vi "Hysteresis-CalculateLinearPosition.vi"(9 "BWD/FWD":T2, 10 "hypothesis":T3(ring)=enum."middle", 11 "relative Range":dbl=1.0) -> (1 "LinBwdFwd":T1)   [LabVIEW 2016]
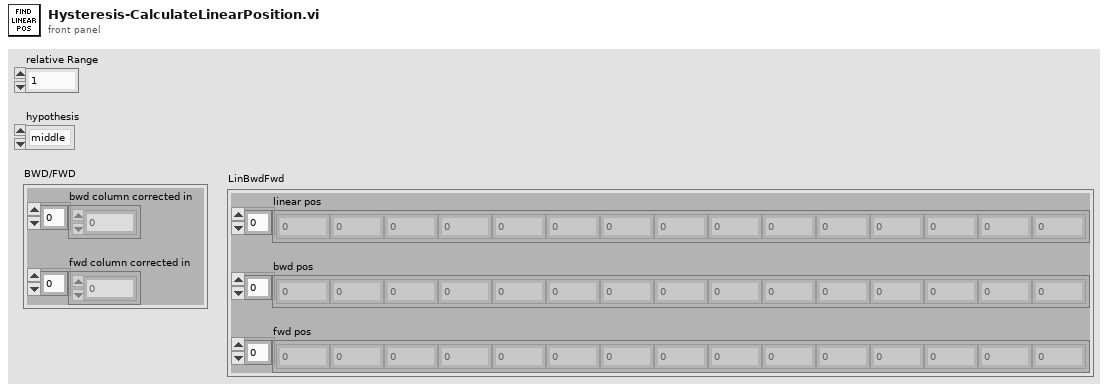
[diagram p1: front panel]
types:
  T1 = cluster{"linear pos ":dbl[], "bwd pos":dbl[], "fwd pos":dbl[]}
  T2 = cluster{"bwd column corrected in":dbl[], "fwd column corrected in":dbl[]}
  T3 = enum16{"bwd", "middle", "fwd", "linear", "2nd esti"}
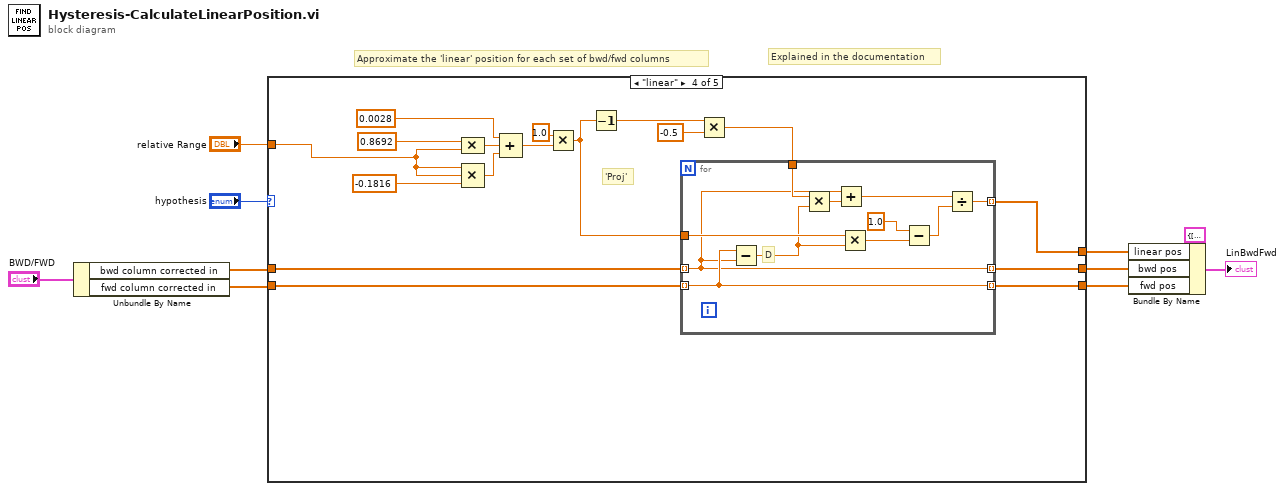
[diagram p0: block diagram]
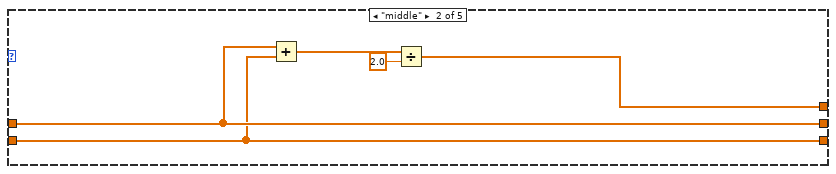
[diagram p3: hidden frame]
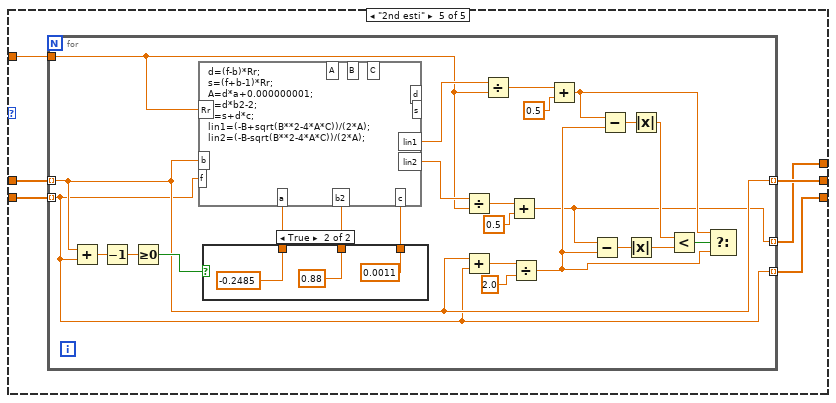
[diagram p5: hidden frame]
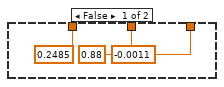
[diagram p6: hidden frame]
diagram:
  # "Explained in the documentation"
  # "Approximate the 'linear' position for each set of bwd/fwd columns"
  n1 = Unbundle By Name("BWD/FWD") -> ("bwd column corrected in"=w6:dbl[], "fwd column corrected in"=w7:dbl[])
  n2 = case shown="\"linear\"" "hypothesis" {
    tunnel: [w11 w14 w19 w36 w48] -> w5
    tunnel: [w12 w16 w19 w34 w50] -> w3
    tunnel: w6 -> [w11 w17 w18 w32 w52]
    tunnel: w7 -> [w12 w16 w19 w33 w53]
    tunnel: [w11 w17 w18 w35 w49] -> w4
    tunnel: "relative Range" -> [_ _ _ w22 w51]
    frame "bwd", Default {
    }
    frame "middle" {
      n3 = Add(x=w17, y=w16) -> (x+y=w15:dbl[])
      n4 = Divide(x=w15, y=2.0) -> (x/y=w14:dbl[])
    }
    frame "fwd" {
    }
    frame "linear" {
      # "'Proj'"
      n5 = Compound Arithmetic op=MULTIPLY(0.8692 ("value"), w22) -> (w31:dbl)
      n6 = Compound Arithmetic op=MULTIPLY(w22, w22, -0.1816 ("value")) -> (w30:dbl)
      n7 = Compound Arithmetic op=ADD(0.0028 ("value"), w31, w30) -> (w24:dbl)
      n8 = Multiply(x=1.0, y=w24) -> (x*y=w20:dbl)
      n9 = Decrement(x=w20) -> (x-1=w26:dbl)
      n10 = Multiply(x=w26, y=-0.5) -> (x*y=w21:dbl)
      n11 = for {
        tunnel: w32 -> [w37] mode=indexing
        tunnel: w33 -> [w38] mode=indexing
        tunnel: w20 -> [w45]
        tunnel: w21 -> [w39]
        tunnel: [w44] -> w36 mode=indexing
        tunnel: [w38] -> w34 mode=indexing
        tunnel: [w37] -> w35 mode=indexing
        # "D"
        n12 = Subtract(x=w38, y=w37) -> (x-y=w40:dbl)
        n13 = Multiply(x=w39, y=w40) -> (x*y=w41:dbl)
        n14 = Add(x=w37, y=w41) -> (x+y=w42:dbl)
        n15 = Multiply(x=w45, y=w40) -> (x*y=w47:dbl)
        n16 = Subtract(x=1.0, y=w47) -> (x-y=w46:dbl)
        n17 = Divide(x=w42, y=w46) -> (x/y=w44:dbl)
      }
    }
    frame "2nd esti" {
      n18 = for {
        tunnel: w53 -> [w57] mode=indexing
        tunnel: w52 -> [w58] mode=indexing
        tunnel: w51 -> [w66]
        tunnel: [w58] -> w49 mode=indexing
        tunnel: [w57] -> w50 mode=indexing
        tunnel: [w54] -> w48 mode=indexing
        n19 = Add(x=w58, y=w57) -> (x+y=w78:dbl)
        n20 = Decrement(x=w78) -> (x-1=w76:dbl)
        n21 = Greater Or Equal To 0?(x=w76) -> (x >= 0?=w77:bool)
        n22 = case shown="True" w77 {
          tunnel: [0.2485 ("input variable") -0.2485 ("input variable")] -> w72
          tunnel: [0.88 ("input variable") 0.88 ("input variable")] -> w71
          tunnel: [-0.0011 ("input variable") 0.0011 ("input variable")] -> w70
          frame False {
          }
          frame True {
          }
        }
        n23 = formula code="d=(f-b)*Rr;\ns=(f+b-1)*Rr;\nA=d*a+0.000000001;\nB=d*b2-2;\nC=s+d*c;\nlin1=(-B+sqrt(B**2-4*A*C))/(2*A);\nlin2=(-B-sqrt(B**2-4*A*C))/(2*A);"("b"=w58, "f"=w57, "Rr"=w66, "a"=w72, "b2"=w71, "c"=w70) -> ("lin1"=w67:dbl, "lin2"=w73:dbl)  [unwired: 5 out]
        n24 = Divide(x=w73, y=w66) -> (x/y=w75:dbl)
        n25 = Add(x=w58, y=w57) -> (x+y=w65:dbl)
        n26 = Divide(x=w67, y=w66) -> (x/y=w68:dbl)
        n27 = Add(x=w75, y=0.5) -> (x+y=w54:dbl)
        n28 = Divide(x=w65, y=2.0) -> (x/y=w56:dbl)
        n29 = Add(x=w68, y=0.5) -> (x+y=w55:dbl)
        n30 = Subtract(x=w54, y=w56) -> (x-y=w62:dbl)
        n31 = Subtract(x=w55, y=w56) -> (x-y=w63:dbl)
        n32 = Absolute Value(x=w62) -> (abs(x)=w61:dbl)
        n33 = Absolute Value(x=w63) -> (abs(x)=w60:dbl)
        n34 = Less?(x=w60, y=w61) -> (x < y?=w59:bool)
        n35 = Select(t=w55, s=w59, f=w56) -> ()  [unwired: 1 out]
      }
    }
  }
  n36 = Bundle By Name(cluster=T1 {"linear pos "=[], "bwd pos"=[], "fwd pos"=[]} ("LinBwdFwd"), "linear pos"=w5, "bwd pos"=w4, "fwd pos"=w3) -> (→"LinBwdFwd":T1)
